vi "update voltage range in ui.vi"(8 "error in (no error)":errorcluster caption="에러 입력(에러 없음)", 10 "voltage range":dbl, 11 "Haptic IC 입력":refnum<class "Haptic IC.lvclass">) -> (0 "error out":errorcluster caption="에러 출력", 3 "Haptic IC 출력":refnum<class "Haptic IC.lvclass">)   [LabVIEW 2020, in "Haptic IC.lvclass"]
uses:
  Haptic IC.lvclass
  Haptic IC.lvclass/Haptic IC.ctl
  Accessors/Read voltage range ref.vi
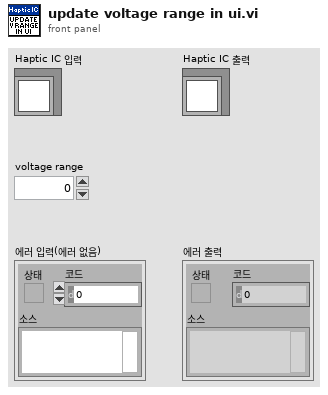
[diagram p1: front panel]
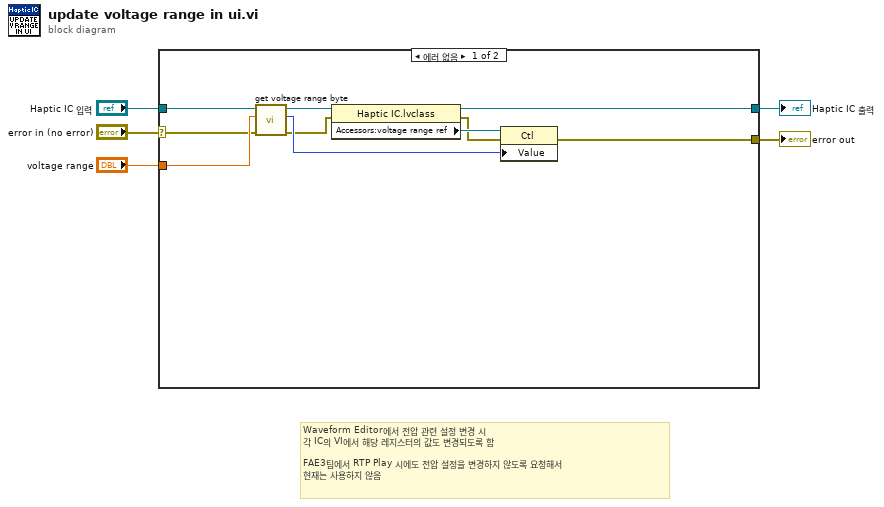
[diagram p0: block diagram]
diagram:
  # "Waveform Editor에서 전압 관련 설정 변경 시\n각 IC의 VI에서 해당 레지스터의 값도 변경되도록 함\n\nFAE3팀에서 RTP Play 시에도 전압 설정을 변경하지 않도록 요청해서\n현재는 사용하지 않음"
  n1 = case shown="에러 없음" "error in (no error)" {
    selector: "error in (no error)" -> [w9 w17]
    tunnel: [w6 w17] -> w4
    tunnel: [w13 w16] -> w2
    tunnel: "Haptic IC 입력" -> [w15 w16]
    tunnel: "voltage range" -> [w11 _]
    frame No Error {
      n2 = call-dynamic "get voltage range byte.vi"("error in (no error)"=w9, "voltage range"=w11, "Haptic IC 입력"=w15) -> ("error out"=w8:errorcluster, "byte value"=w10:u8, "Haptic IC 출력"=w14:refnum<class "Haptic IC.lvclass">)  [unwired: 6 in]
      n3 = property class="Haptic IC.lvclass"(reference=w14, error in=w8) -> (reference out=w13:refnum<class "Haptic IC.lvclass">, error out=w7:errorcluster, "Accessors:voltage range ref"=w12:refnum<vi>)
      n4 = property class="Ctl"(reference=w12, error in=w7, "Value"=w10) -> (error out=w6:errorcluster)  [unwired: 1 out]
    }
    frame Error {
    }
  }
  "error out" <- w4
  "Haptic IC 출력" <- w2
